vi "Laser_COM_v2.vi"() -> ()   [LabVIEW 2014]
uses:
  <vilib>/Instr/_visa.llb/Select Event Type.ctl
  <vilib>/Instr/_visa.llb/VISA Configure Serial Port (Instr).vi
panel:
  out "7":bool
  out "6":bool
  out "4":bool
  out "5":bool
  out "3":bool
  out "2":bool
  out "1":bool
  out "0":bool
  in  "Control PL":bool
  in  "Control GL":bool
  out "DB25 ML":bool
  out "RS232 ML":bool
  in  "Control ML":bool
  out "on/off? 5":bool
  in  "Laser":bool
  out "Laser EM":bool caption="Излучение включено!"
  out "on/off? 3":bool
  out "on/off? 2":bool
  in  "Send":bool
  in  "write buffer":string caption="Передать команду"
  out "COM_connect":bool
  in  "Connect":bool
  out "SN:":string
  out "ID:":string
  out "Guide  laser":bool
  out "module temp":dbl caption="Темп. модуля" format="%#_g °C"
  in  "Power":dbl(slide) caption="Мощность излучения, %" min=0.0 max=100.0 step=0.5 scale=0.0..100.0 scale format="%#.2g"
  in  "Laser pilot":bool caption="Лазер пилот"
  in  "COM":refnum<visa-resource-name>="COM1" caption="Laser COM-port"
  out "read buffer":string caption="ОТВЕТ:"
  out "error out":errorcluster
  in  "error in (no error)":errorcluster
  # "ID:\n\nSN:"
  # "Блок  управления основным лазером"
  # "RS-232"
  # "DB-25"
  # "T модуля -"
  # "RS-232"
  # "Мощьность  излучения, %"
  # "DB-25"
  # "DB-25"
  # "Пилот Лазер"
  # "RS-232"
  # "DB-25"
  # "Терминал"
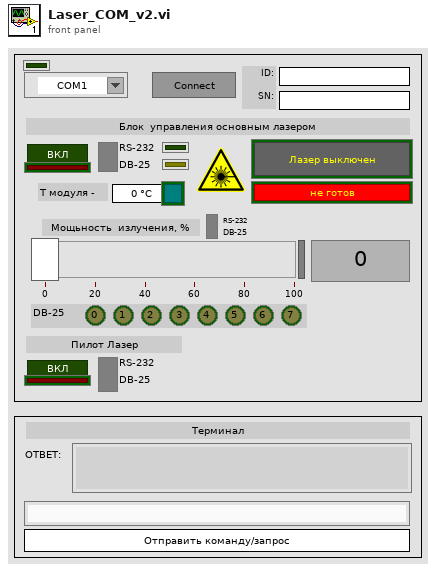
[diagram p1: front panel]
types:
  T1 = typedef "Select Event Type.ctl" = u32
  T2 = cluster{"Power control by DB-25":bool, "Reserved[1]":bool, "AuxOFF control by DB-25":bool, "Guide laser control by DB-25":bool, "Reserved[4]":bool, "Reserved[5]":bool, "Reserved[6]":bool, "Emission Modulation control by DB-25":bool, "The laser is in Jump PRR mode":bool, "Reserved[9]":bool, "Bitstream 1 (BS1) mode is active":bool, "Reserved[11]":bool, "PRR controlled by Sync line in DB-25":bool, "Emission Enable control by DB-25":bool, "APD mode is controlled by DB-25":bool, "Automatic latch":bool, "Reserved[16]":bool, "Reserved[17]":bool, "Reserved[18]":bool, "The laser is in Sweep PRR mode":bool, "The laser is in Follow PRR mode":bool, "Manual Prepump mode is active":bool, "Manual residual is controlled by DB-25":bool, "Reserved[23]":bool, "Reserved[24]":bool, "Guide laser safety function is not activated":bool, "Discharge circuit safety function is activated":bool, "Reserved[27]":bool, "Reserved[28]":bool, "Reserved[29]":bool, "Reserved[30]":bool, "Reserved[31]":bool}
  T3 = cluster{"Rack  reflection":bool, "Temp Laser module":bool, "Temp Laser head":bool, "System Alarm":bool, "+24V main supply Alarm":bool, "HK supply  Alarm":bool, "Laser ready":bool, "Warning is activated":bool}
  T4 = cluster{"Emergency stop":bool, "External PRR [1]":bool, "External PRR [2]":bool, "Reserved [3]":bool, "Reserved [4]":bool, "Guide laser":bool, "Reserved [6]":bool, "Reserved [7]":bool, "Laser emission":bool, "Reserved [9]":bool, "Reserved [10]":bool, "Laser emission command was received by RS-232":bool, "Guide laser command was received by RS-232":bool, "24V Main supply voltage is in specified range":bool, "HK supply voltage is in specified range":bool, "Emission Enable is switched by RS-232":bool, "Reserved [16]":bool, "Reserved [17]":bool, "Reserved [18]":bool, "Reserved [19]":bool, "Reserved [20]":bool, "Reserved [21]":bool, "Reserved [22]":bool, "Reserved [23]":bool, "Reserved [24]":bool, "Reserved [25]":bool, "Reserved [26]":bool, "Reserved [27]":bool, "Reserved [28]":bool, "Reserved [29]":bool, "Reserved [30]":bool, "Reserved [31]":bool}
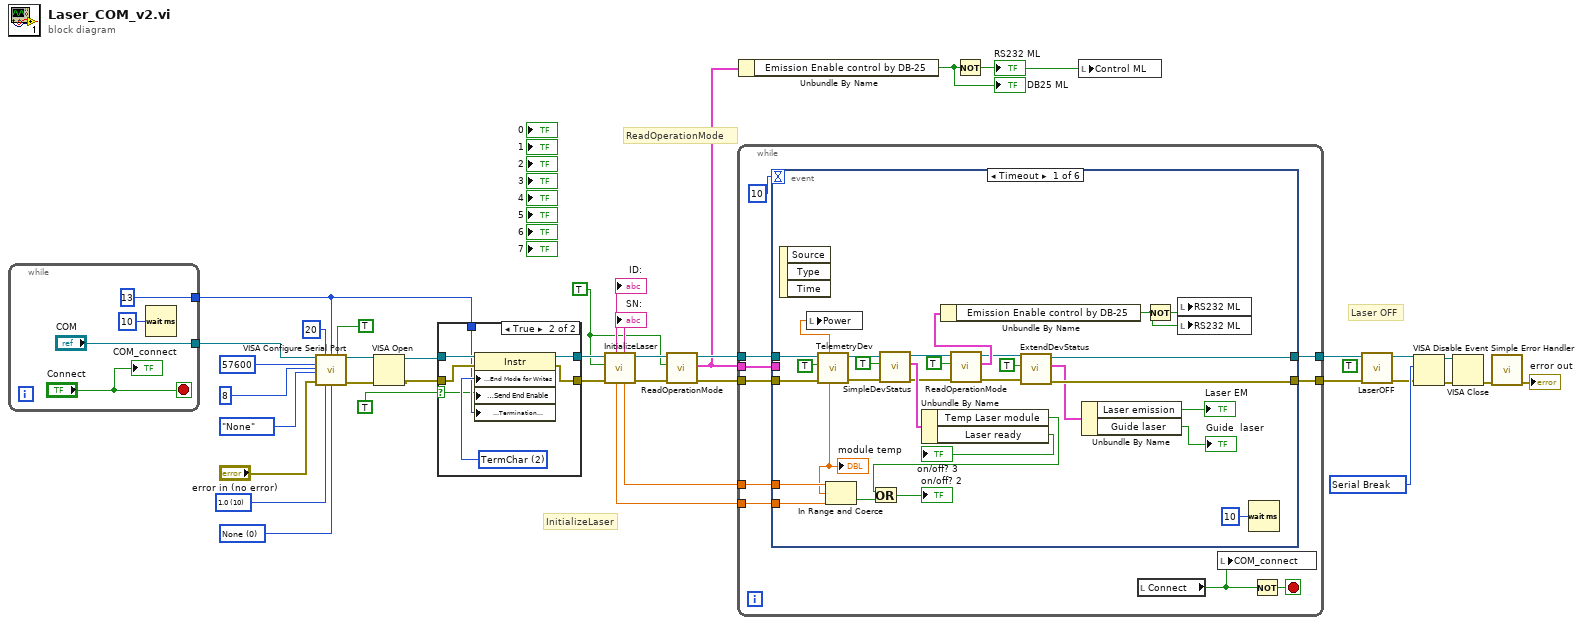
[diagram p0: block diagram]
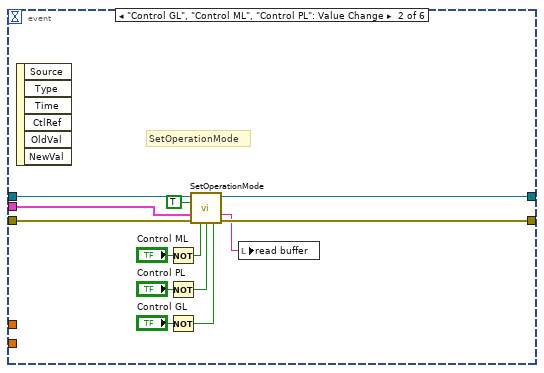
[diagram p2: hidden frame]
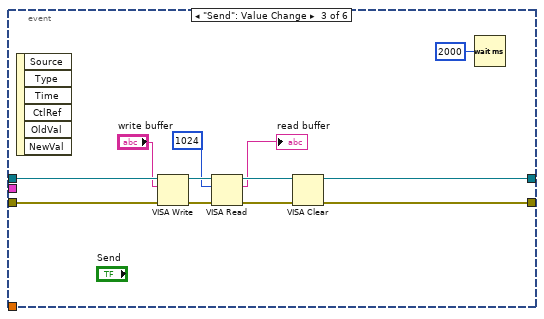
[diagram p3: hidden frame]
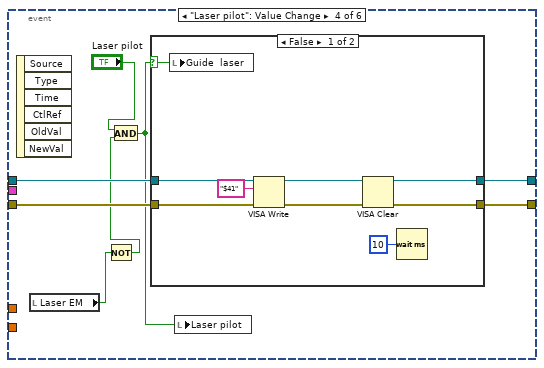
[diagram p4: hidden frame]
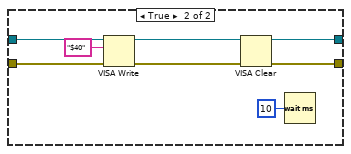
[diagram p5: hidden frame]
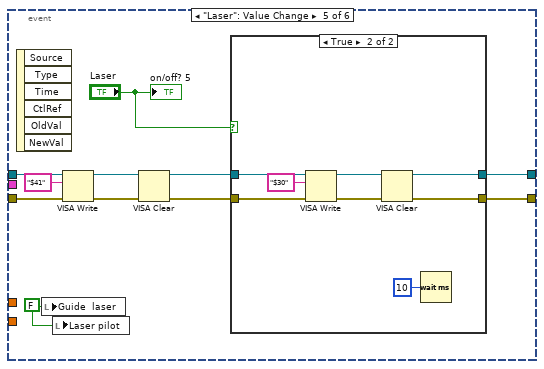
[diagram p6: hidden frame]
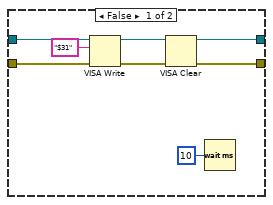
[diagram p7: hidden frame]
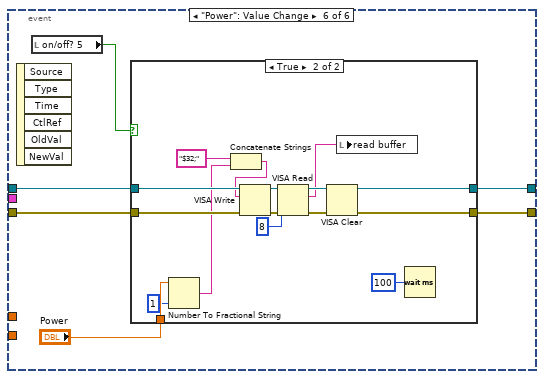
[diagram p8: hidden frame]
diagram:
  w19 = T1 1073684515 items=["Service Request"=1073684491, "Trigger"=3221168138, "Clear"=1073684493, "VXI Signal"=1073684512, "VXI/VME Interrupt"=3221168161, "VXI/VME Sysfail"=1073684509, "VXI/VME Sysreset"=1073684510, "GPIB CIC"=1073684498, "GPIB Talk"=1073684499, "GPIB Listen"=1073684500, "PXI Interrupt"=1073684514, "Serial Break"=1073684515, "Serial TermChar"=1073684516, "Serial CTS"=1073684521, "Serial DSR"=1073684522, "Serial DCD"=1073684524, "Serial RI"=1073684526, "Serial Character"=1073684533, "USB Interrupt"=1073684535, "All Enabled"=1073709055] ("Event Type")
  (unwired) TRUE
  w24 = u16 0 items=["None", "XON/XOFF", "RTS/CTS", "XON/XOFF & RTS/CTS", "DTR/DSR", "XON/XOFF & DTR/DSR"] ("flow control (0:none)")
  w6 = TRUE
  w31 = u16 10 items=["1.0"=10, "1.5"=15, "2.0"=20] ("stop bits (10: 1 bit)")
  # "Laser OFF"
  # "ReadOperationMode"
  # "InitializeLaser"
  n1 = while {
    tunnel: ["COM"] -> w23
    tunnel: [i16 13 ("term_char")] -> w22
    stop <- "Connect" stop-if-true
    n2 = Wait (ms)(milliseconds to wait=u32 10) -> ()  [unwired: 1 out]
    "COM_connect" <- "Connect"
  }
  n3 = call-poly "VISA Configure Serial Port"("VISA resource name"=w23, "timeout (10sec)"=u32 20, "termination char\n(0xA = '\\n' = LF)"=w22, "Enable Termination\nChar (T)"=TRUE ("Enable Termination\nChar (T)"), "baud rate (9600)"=u32 57600 ("baud rate"), "data bits (8)"=u16 8, "parity (0:none)"=enum16{"None", "Odd", "Even", "Mark", "Space"}."None", "error in (no error)"="error in (no error)", "stop bits (10: 1 bit)"=w31, "flow control (0:none)"=w24) -> ("VISA resource name out"=w34:refnum<visa-resource-name>, "error out"=w33:errorcluster)  [unwired: 4 in]
  n4 = VISA Open(error in (no error)=w33, VISA resource name=w34) -> (VISA resource name=w28:refnum<visa-resource-name>, error out=w29:errorcluster)  [unwired: 3 in]
  n5 = case shown="True" TRUE ("End write with termination character?") {
    selector: TRUE ("End write with termination character?") -> [_ w45]
    tunnel: w28 -> [w43 w51]
    tunnel: w29 -> [w44 w50]
    tunnel: [w43 w49] -> w17
    tunnel: [w44 w48] -> w18
    tunnel: w22 -> [_ w46]
    frame False {
    }
    frame True {
      w47 = u16 2 items=["None", "LastBit", "TermChar", "Break"] ("Serial Settings:Serial End Mode for Writes")
      n6 = property class="Instr"(reference=w51, error in=w50, "Serial Settings:End Mode for Writes"=w47, "Message Based Settings:Send End Enable"=w45, "Message Based Settings:Termination Character"=w46) -> (reference out=w49:refnum<visa-resource-name>, error out=w48:errorcluster)
    }
  }
  n7 = call "InitializeLaser.vi"("error in"=w18, "ON/OFF"=w6, "VISA resource name in"=w17) -> ("error out"=w7:errorcluster, "VISA resource name out"=w8:refnum<visa-resource-name>, "Tmax"=w16:dbl, "SN:"=→"SN:":string, "Tmin"=w15:dbl, "Лазер: ID:"=→"ID:":string)  [unwired: 1 in, 2 out]
  n8 = call "ReadOperationMode.vi"("error in"=w7, "ON/OFF"=w6, "VISA resource name in"=w8) -> ("error out"=w9:errorcluster, "Operation Mode Status"=w3:T2, "VISA resource name out"=w10:refnum<visa-resource-name>)  [unwired: 5 in, 1 out]
  n9 = while {
    tunnel: w9 -> [w56]
    tunnel: w10 -> [w57]
    tunnel: [w59] -> w12
    tunnel: [w58] -> w11
    tunnel: w16 -> [w54]
    tunnel: w15 -> [w53]
    tunnel: w3 -> [w52]
    stop <- w61 stop-if-true
    n10 = event shown="[0] Timeout" {
      selector: _ -> [_ _ _ _ _ _]
      dyn-events: _ -> [_ _ _ _ _ _]
      timeout: 10 -> [_ _ _ _ _ _]
      tunnel: w57 -> [w70 w104 w116 w124 w151 w173]
      tunnel: w56 -> [w69 w103 w115 w123 w150 w172]
      tunnel: [w74 w101 w110 w122 w146 w171] -> w59
      tunnel: [w73 w102 w109 w121 w145 w170] -> w58
      tunnel: w53 -> [w89 _ _ _ _ _]
      tunnel: w54 -> [w90 _ _ _ _ _]
      tunnel: w52 -> [_ w98 _ _ _ _]
      event Timeout {
        n11 = event-data() -> ()  [unwired: 1 in, 3 out]
        n12 = call "TelemetryDev.vi"("error in"=w69, "ON/OFF"=TRUE, "VISA resource name in"=w70) -> ("error out"=w66:errorcluster, "VISA resource name out"=w67:refnum<visa-resource-name>, "module temp"=w65:dbl, "Laser Power,%"=w64:dbl)  [unwired: 4 in, 1 out]
        "module temp" <- w65
        n13 = local write "Power"(w64) -> ()
        n14 = In Range and Coerce(upper limit=w90, x=w65, lower limit=w89) -> (In Range?=w77:bool)  [unwired: 1 out]
        n15 = call "SimpleDevStatus.vi"("error in"=w66, "ON/OFF"=TRUE ("Boolean"), "VISA resource name in"=w67) -> ("error out"=w82:errorcluster, "Device Status"=w85:T3, "VISA resource name out"=w83:refnum<visa-resource-name>)  [unwired: 5 in]
        n16 = Unbundle By Name(w85) -> ("Temp Laser module"=w87:bool, "Laser ready"=→"on/off? 3":bool)
        n17 = Or(x=w87, y=w77) -> (x .or. y?=→"on/off? 2":bool)
        n18 = call "ReadOperationMode.vi"("error in"=w82, "ON/OFF"=TRUE, "VISA resource name in"=w83) -> ("error out"=w75:errorcluster, "Operation Mode Status"=w80:T2, "VISA resource name out"=w76:refnum<visa-resource-name>)  [unwired: 5 in, 1 out]
        n19 = Unbundle By Name(w80) -> ("Emission Enable control by DB-25"=w78:bool)
        n20 = call "ExtendDevStatus.vi"("error in"=w75, "ON/OFF"=TRUE, "VISA resource name in"=w76) -> ("error out"=w73:errorcluster, "Extend Device Status"=w71:T4, "VISA resource name out"=w74:refnum<visa-resource-name>)  [unwired: 5 in]
        n21 = Unbundle By Name(w71) -> ("Laser emission"=→"Laser EM":bool, "Guide laser"=→"Guide  laser":bool)
        n22 = Not(x=w78) -> (.not. x?=w79:bool)
        n23 = local write "RS232 ML"(w79) -> ()
        n24 = local write "RS232 ML"(w78) -> ()
        n25 = Wait (ms)(milliseconds to wait=u32 10) -> ()  [unwired: 1 out]
      }
      event "Control GL", "Control ML", "Control PL": Value Change {
        # "SetOperationMode"
        n26 = event-data() -> ()  [unwired: 1 in, 6 out]
        n27 = Not(x="Control ML") -> (.not. x?=w93:bool)
        n28 = Not(x="Control PL") -> (.not. x?=w92:bool)
        n29 = Not(x="Control GL") -> (.not. x?=w96:bool)
        n30 = call "SetOperationMode.vi"("VISA resource name in"=w104, "ON/OFF"=TRUE, "Operation Mode Status"=w98, "error in"=w103, "Laser"=w93, "Power"=w92, "Guide laser"=w96) -> ("VISA resource name out"=w101:refnum<visa-resource-name>, "Message"=w99:string, "error out"=w102:errorcluster)  [unwired: 6 in]
        n31 = local write "read buffer"(w99) -> ()
      }
      event "Send": Value Change {
        n32 = event-data() -> ()  [unwired: 1 in, 6 out]
        n33 = VISA Write(VISA resource name=w116, write buffer="write buffer", error in (no error)=w115) -> (VISA resource name out=w114:refnum<visa-resource-name>, error out=w113:errorcluster)  [unwired: 1 out]
        n34 = VISA Read(VISA resource name=w114, byte count=u32 1024, error in (no error)=w113) -> (VISA resource name out=w112:refnum<visa-resource-name>, read buffer=→"read buffer":string, error out=w111:errorcluster)  [unwired: 1 out]
        n35 = VISA Clear(VISA resource name=w112, error in (no error)=w111) -> (VISA resource name out=w110:refnum<visa-resource-name>, error out=w109:errorcluster)
        n36 = Wait (ms)(milliseconds to wait=u32 2000) -> ()  [unwired: 1 out]
      }
      event "Laser pilot": Value Change {
        n37 = event-data() -> ()  [unwired: 1 in, 6 out]
        n38 = local read "Laser EM"() -> (w120:bool)
        n39 = Not(x=w120) -> (.not. x?=w118:bool)
        n40 = And(x="Laser pilot", y=w118) -> (x .and. y?=w117:bool)
        n41 = case shown="False" w117 {
          selector: w117 -> [w131 _]
          tunnel: w124 -> [w133 w141]
          tunnel: w123 -> [w132 w140]
          tunnel: [w128 w137] -> w122
          tunnel: [w127 w136] -> w121
          frame False {
            n42 = local write "Guide  laser"(w131) -> ()
            n43 = VISA Write(VISA resource name=w133, write buffer="$41", error in (no error)=w132) -> (VISA resource name out=w126:refnum<visa-resource-name>, error out=w125:errorcluster)  [unwired: 1 out]
            n44 = VISA Clear(VISA resource name=w126, error in (no error)=w125) -> (VISA resource name out=w128:refnum<visa-resource-name>, error out=w127:errorcluster)
            n45 = Wait (ms)(milliseconds to wait=u32 10 ("millisecond multiple")) -> ()  [unwired: 1 out]
          }
          frame True {
            n46 = VISA Write(VISA resource name=w141, write buffer="$40", error in (no error)=w140) -> (VISA resource name out=w135:refnum<visa-resource-name>, error out=w134:errorcluster)  [unwired: 1 out]
            n47 = VISA Clear(VISA resource name=w135, error in (no error)=w134) -> (VISA resource name out=w137:refnum<visa-resource-name>, error out=w136:errorcluster)
            n48 = Wait (ms)(milliseconds to wait=u32 10 ("millisecond multiple")) -> ()  [unwired: 1 out]
          }
        }
        n49 = local write "Laser pilot"(w117) -> ()
      }
      event "Laser": Value Change {
        w144 = FALSE ("on/off?")
        n50 = event-data() -> ()  [unwired: 1 in, 6 out]
        n51 = local write "Guide  laser"(w144) -> ()
        n52 = local write "Laser pilot"(w144) -> ()
        n53 = VISA Write(VISA resource name=w151, write buffer="$41", error in (no error)=w150) -> (VISA resource name out=w143:refnum<visa-resource-name>, error out=w142:errorcluster)  [unwired: 1 out]
        n54 = VISA Clear(VISA resource name=w143, error in (no error)=w142) -> (VISA resource name out=w148:refnum<visa-resource-name>, error out=w147:errorcluster)
        n55 = case shown="True" "Laser" {
          tunnel: w148 -> [w159 w167]
          tunnel: w147 -> [w158 w166]
          tunnel: [w157 w165] -> w146
          tunnel: [w156 w164] -> w145
          frame False {
            n56 = VISA Write(VISA resource name=w159, write buffer="$31", error in (no error)=w158) -> (VISA resource name out=w153:refnum<visa-resource-name>, error out=w154:errorcluster)  [unwired: 1 out]
            n57 = VISA Clear(VISA resource name=w153, error in (no error)=w154) -> (VISA resource name out=w157:refnum<visa-resource-name>, error out=w156:errorcluster)
            n58 = Wait (ms)(milliseconds to wait=u32 10) -> ()  [unwired: 1 out]
          }
          frame True {
            n59 = VISA Write(VISA resource name=w167, write buffer="$30", error in (no error)=w166) -> (VISA resource name out=w162:refnum<visa-resource-name>, error out=w161:errorcluster)  [unwired: 1 out]
            n60 = VISA Clear(VISA resource name=w162, error in (no error)=w161) -> (VISA resource name out=w165:refnum<visa-resource-name>, error out=w164:errorcluster)
            n61 = Wait (ms)(milliseconds to wait=u32 10) -> ()  [unwired: 1 out]
          }
        }
        "on/off? 5" <- "Laser"
      }
      event "Power": Value Change {
        n62 = event-data() -> ()  [unwired: 1 in, 6 out]
        n63 = local read "on/off? 5"() -> (w174:bool)
        n64 = case shown="True" w174 {
          tunnel: w173 -> [w176 w188]
          tunnel: w172 -> [w175 w187]
          tunnel: [w176 w186] -> w171
          tunnel: [w175 w185] -> w170
          tunnel: "Power" -> [_ w182]
          frame False {
          }
          frame True {
            n65 = Number To Fractional String(number=w182, precision (6)=i16 1) -> (F-format string=w181:string)  [unwired: 2 in]
            n66 = Concatenate Strings("$32;" ("write buffer"), w181) -> (w183:string)
            n67 = VISA Write(VISA resource name=w188, write buffer=w183, error in (no error)=w187) -> (VISA resource name out=w190:refnum<visa-resource-name>, error out=w189:errorcluster)  [unwired: 1 out]
            n68 = VISA Read(VISA resource name=w190, byte count=u32 8, error in (no error)=w189) -> (VISA resource name out=w191:refnum<visa-resource-name>, read buffer=w178:string, error out=w192:errorcluster)  [unwired: 1 out]
            n69 = VISA Clear(VISA resource name=w191, error in (no error)=w192) -> (VISA resource name out=w186:refnum<visa-resource-name>, error out=w185:errorcluster)
            n70 = local write "read buffer"(w178) -> ()
            n71 = Wait (ms)(milliseconds to wait=u32 100) -> ()  [unwired: 1 out]
          }
        }
      }
    }
    n72 = local read "Connect"() -> (w60:bool)
    n73 = local write "COM_connect"(w60) -> ()
    n74 = Not(x=w60) -> (.not. x?=w61:bool)
  }
  n75 = Unbundle By Name(w3) -> ("Emission Enable control by DB-25"=w4:bool)
  "DB25 ML" <- w4
  n76 = Not(x=w4) -> (.not. x?=w5:bool)
  "RS232 ML" <- w5
  n77 = local write "Control ML"(w5) -> ()
  n78 = call "LaserOFF.vi"("error in"=w11, "VISA resource name in"=w12) -> ("error out"=w1:errorcluster, "VISA resource name out"=w2:refnum<visa-resource-name>)  [unwired: 8 in]
  n79 = VISA Disable Event(8:w1, 10:w19, 11:w2) -> (0:w20:errorcluster, 3:w21:refnum<visa-resource-name>)  [unwired: 1 out]
  n80 = VISA Close(VISA resource name=w21, error in (no error)=w20) -> (error out=w25:errorcluster)
  n81 = call <vilib>:"Simple Error Handler.vi"("error in (no error)"=w25) -> ("error out"=→"error out":errorcluster)  [unwired: 4 in, 4 out]
